vi "TDS Make Connection.vi"(8 "error in (no error)":errorcluster, 9 "State":bool, 10 "Connection Configuration":string="DSG30", 11 "Address":string) -> (0 "error out":errorcluster)   [LabVIEW 2025, in "Interface Functions.lvlib"]
uses:
  Interface Functions.lvlib
panel:
  # "Make Connection"
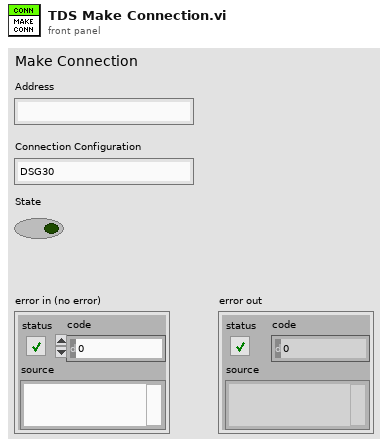
[diagram p1: front panel]
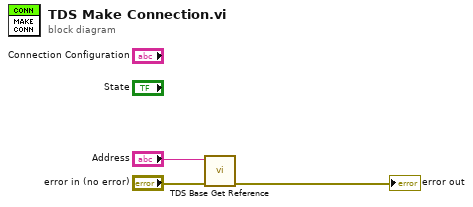
[diagram p0: block diagram]
diagram:
  n1 = call "TDS Base Get Reference.vi"("error in (no error)"="error in (no error)", "Address"="Address") -> ("error out"=→"error out":errorcluster)  [unwired: 8 in, 1 out]
